vi "Argparser AE.vi"(8 "error in (no error)":errorcluster, 11 "LV Argument Parser in":refnum<class "LV Argument Parser.lvclass">) -> (0 "error out":errorcluster, 3 "LV Argument Parser out":refnum<class "LV Argument Parser.lvclass">)   [LabVIEW 2023, in "LV ArgParse.lvlib" / "LV Argument Parser.lvclass"]
uses:
  LV Argument Parser.lvclass
  LV Argument Parser.lvclass/LV Argument Parser.ctl
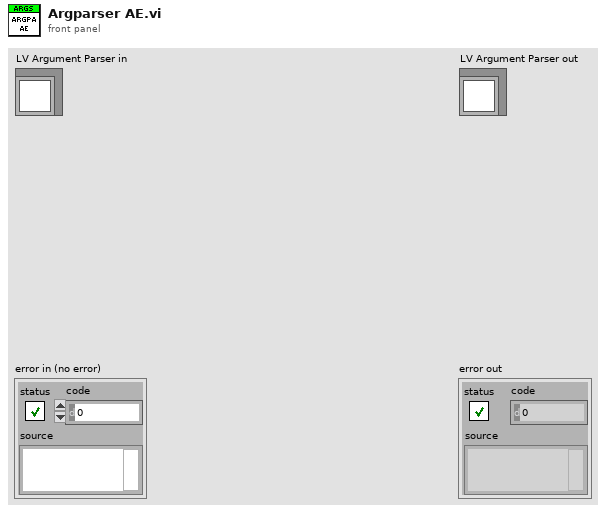
[diagram p1: front panel]
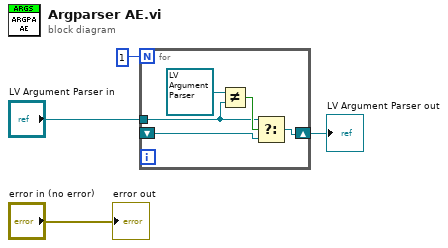
[diagram p0: block diagram]
diagram:
  n1 = for {
    N: 1 -> [_]
    shift-right: [w8] -> w3
    shift-left: _ -> [w9]
    tunnel: "LV Argument Parser in" -> [w5]
    n2 = Not Equal?(x=refnum<class "LV Argument Parser.lvclass"> refnum, y=w5) -> (x != y?=w6:bool)
    n3 = Select(t=w5, s=w6, f=w9) -> (s? t:f=w8:refnum<class "LV Argument Parser.lvclass">)
  }
  "LV Argument Parser out" <- w3
  "error out" <- "error in (no error)"
